vi "Try Match Response.vi"(8 "error in":errorcluster, 10 "ICAN CC Frame":refnum<class "ICAN CC Frame.lvclass">, 11 "Block Upload Transfer in":refnum<class "Block Upload Sub-Block Transfer.lvclass">) -> (0 "error out":errorcluster, 2 "Match":bool, 3 "SDO Transfer out":refnum<class "SDO Transfer.lvclass">)   [LabVIEW 2020, in "CANopen.lvlib" / "SDO Manager.lvlib" / "Block Upload Sub-Block Transfer.lvclass"]
uses:
  Block Upload Sub-Block Transfer.lvclass
  D:/git/CANopen-LabVIEW/source/SDO/SDO Manager/SDO Transfer/SDO Transfer.lvclass
  SDO Transfer/SDO Transfer.lvclass
  HAL/Source/Interfaces/ICAN CC Frame/ICAN CC Frame.lvclass
  D:/git/HAL/Source/Interfaces/IMessage/IMessage.lvclass
  SDO Transfer/SDO Transfer.lvclass/SDO Transfer.ctl
  Block Upload Sub-Block Transfer.lvclass/Block Upload Sub-Block Transfer.ctl
  Block Upload End Transfer/Block Upload End Transfer.lvclass
  HAL/Source/Interfaces/ICommunicate/ICommunicate.lvclass
  CANopen Message/CANopen Message.lvclass
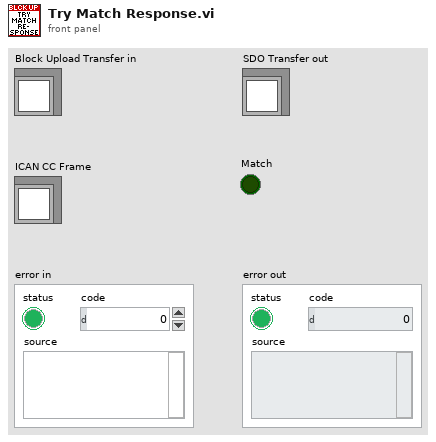
[diagram p1: front panel]
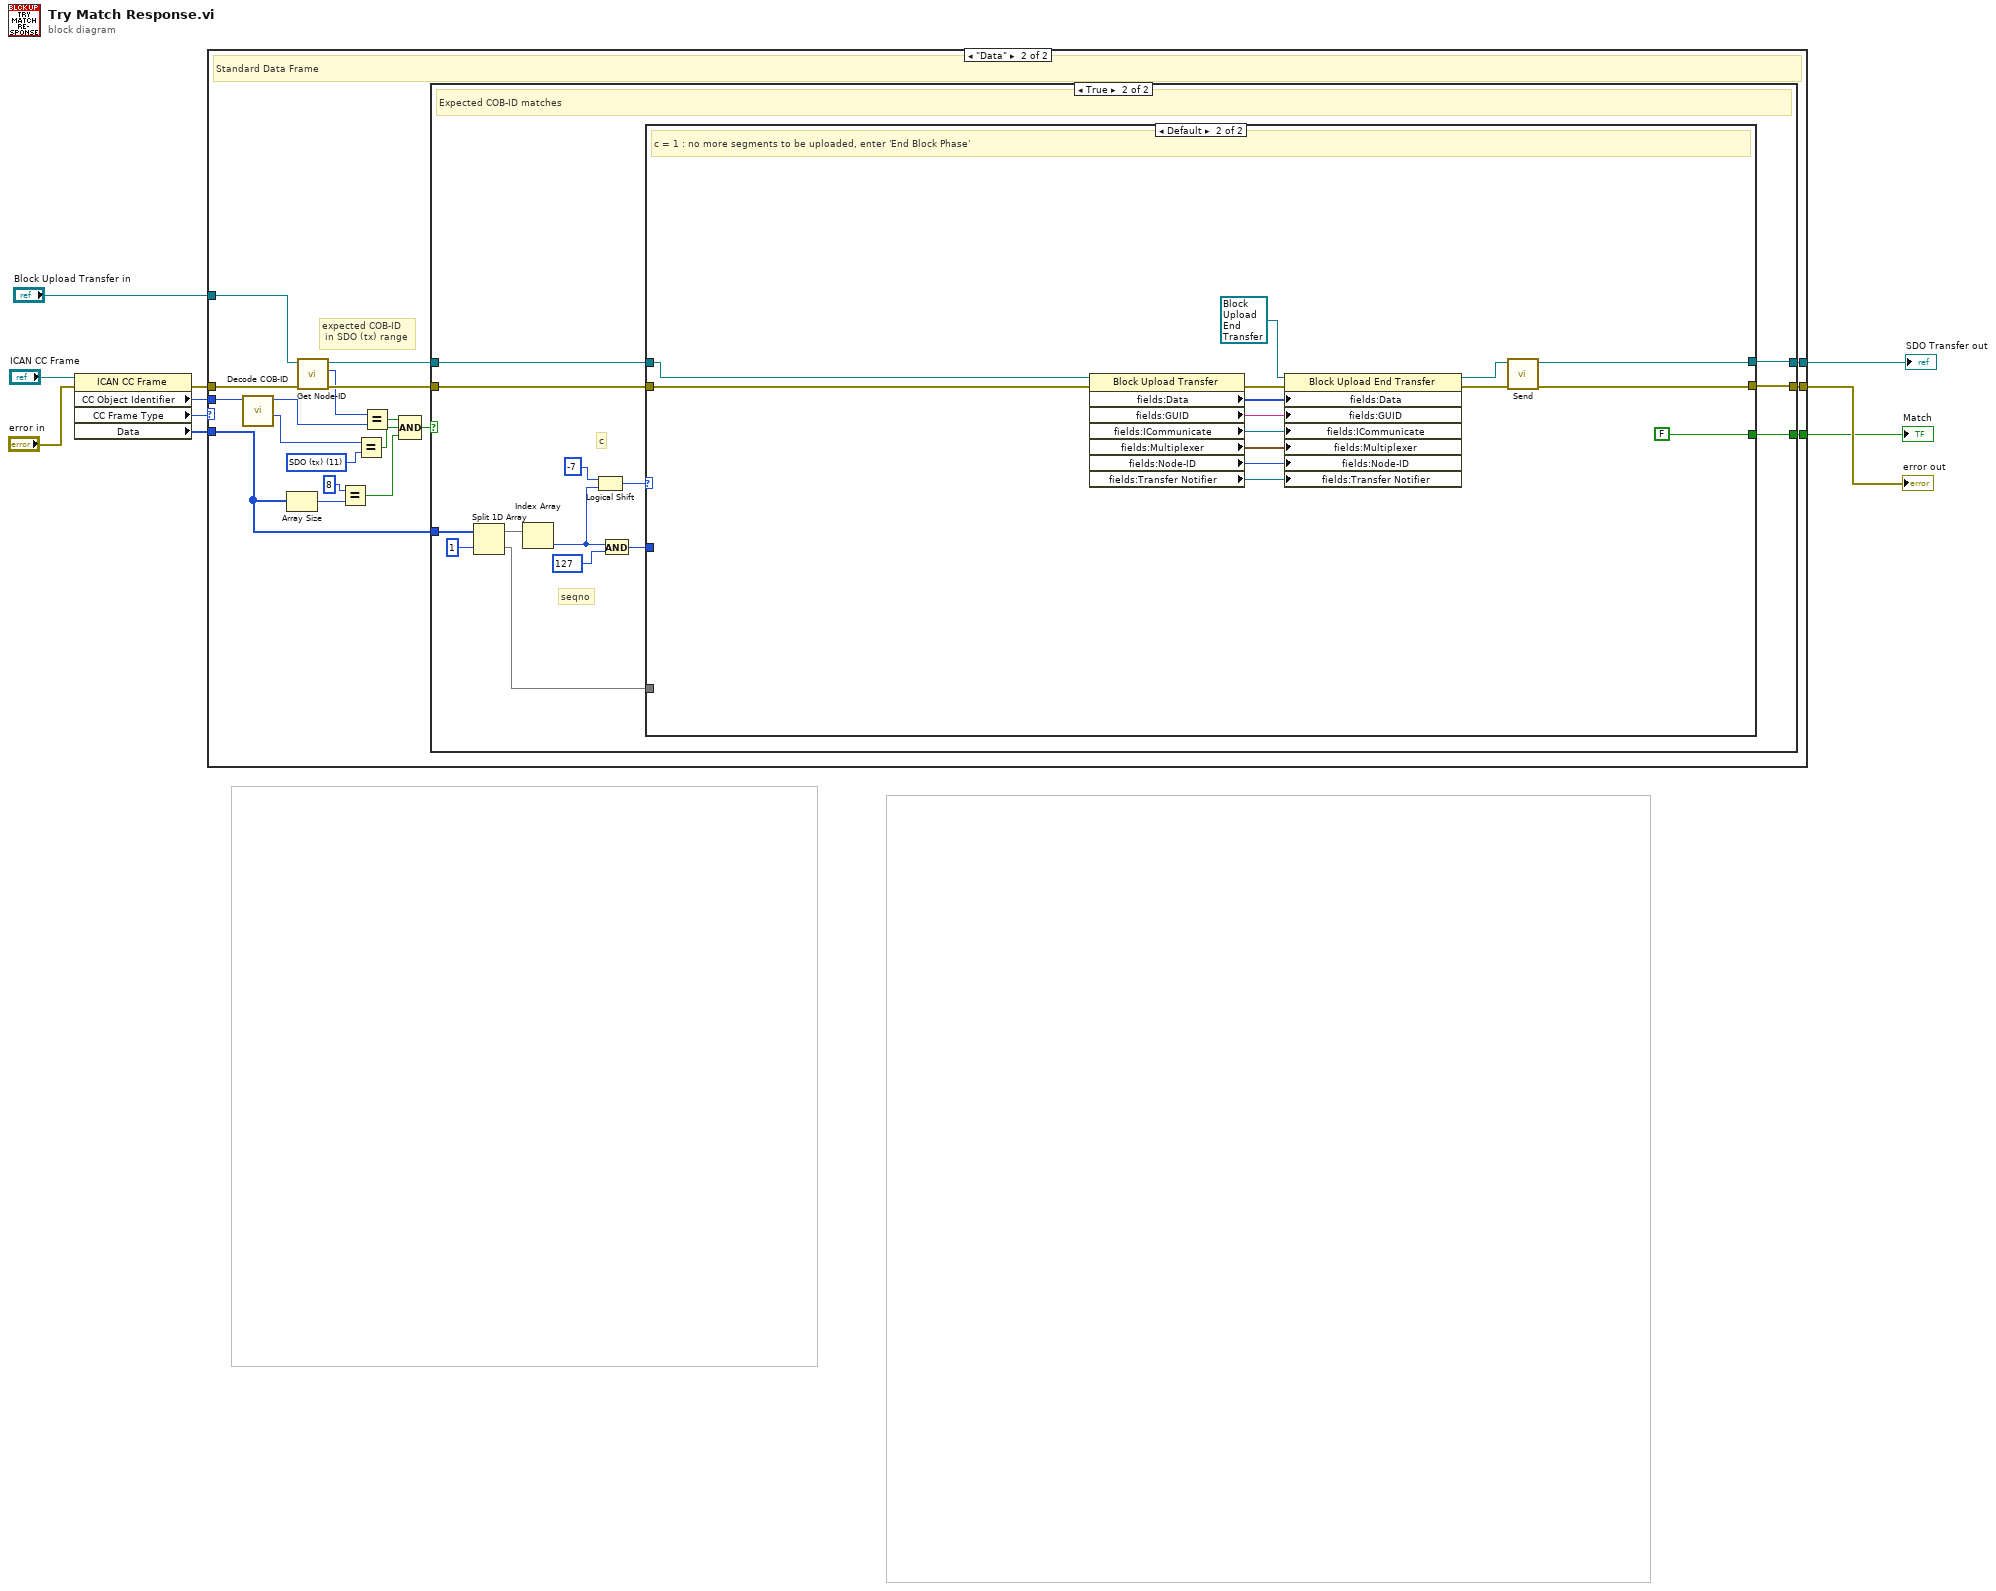
[diagram p0: block diagram]
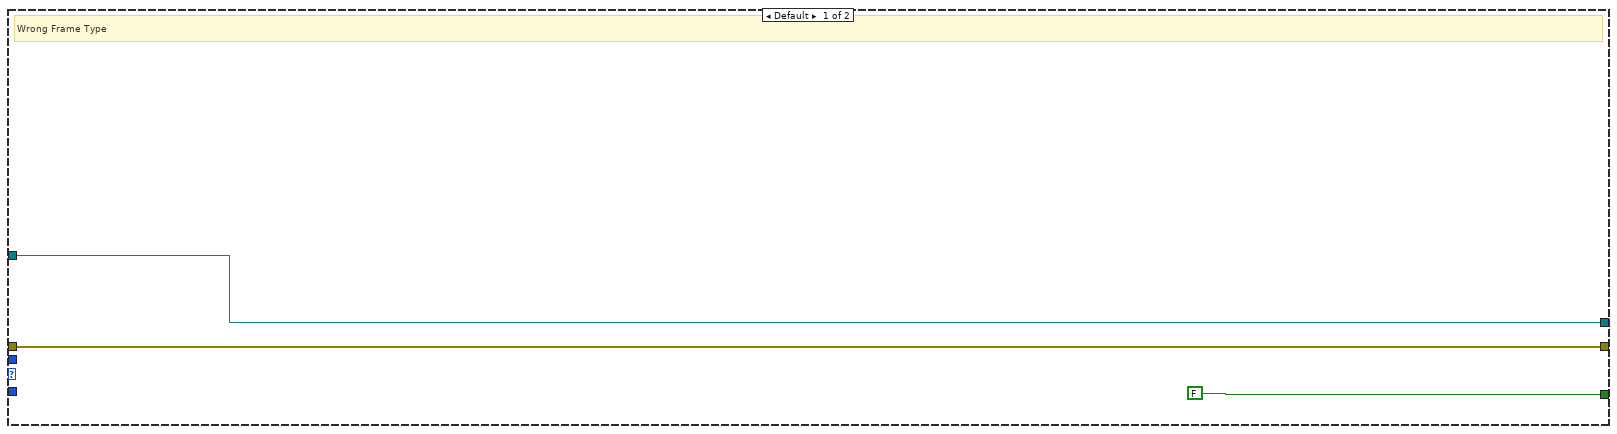
[diagram p2: hidden frame]
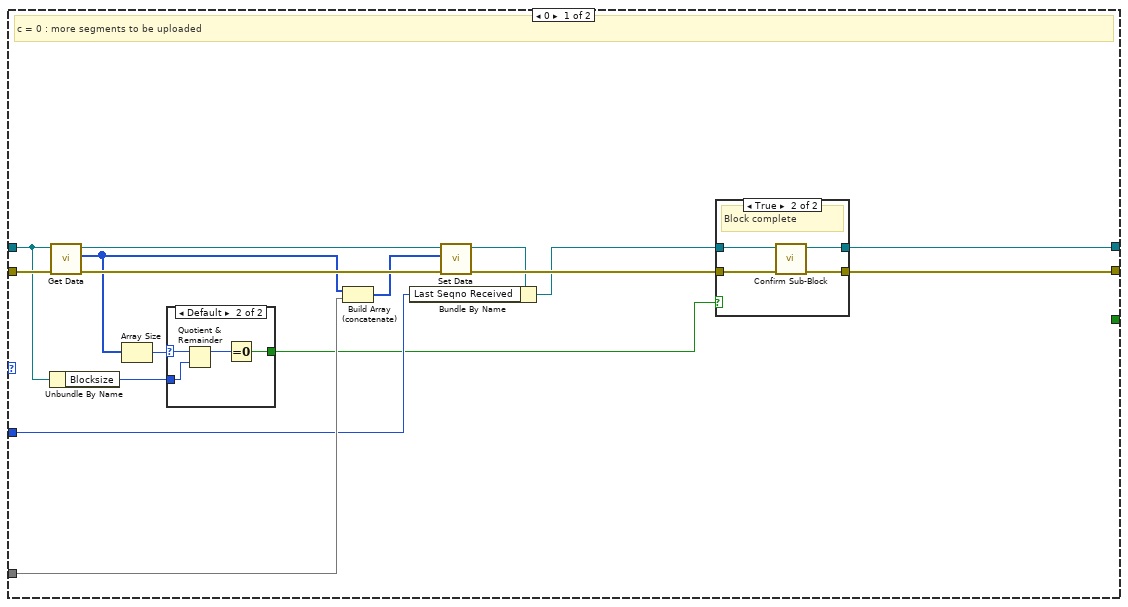
[diagram p4: hidden frame]
diagram:
  n1 = property class="ICAN CC Frame"(reference="ICAN CC Frame", error in="error in") -> (error out=w9:errorcluster, "CC Object Identifier"=w8:u32, "CC Frame Type"=w6:enum8{"Data", "Remote", "Error", "Overload"}, "Data"=w7:u8[])  [unwired: 1 out]
  n2 = case shown="\"Data\"" w6 {
    tunnel: w9 -> [w12 w32]
    tunnel: "Block Upload Transfer in" -> [w11 w31]
    tunnel: [w11 w28] -> w2
    tunnel: [w12 w27] -> w10
    tunnel: [FALSE w26] -> w1
    tunnel: w8 -> [_ w25]
    tunnel: w7 -> [_ w14]
    frame Default {
      # "Wrong Frame Type"
    }
    frame "Data" {
      w22 = u8 11 items=["NMT"=0, "EMCY/SYNC"=1, "TIME"=2, "PDO1 (tx)"=3, "PDO1 (rx)"=4, "PDO2 (tx)"=5, "PDO2 (rx)"=6, "PDO3 (tx)"=7, "PDO3 (rx)"=8, "PDO4 (tx)"=9, "PDO4 (rx)"=10, "SDO (tx)"=11, "SDO (rx)"=12, "NMT error control"=14] ("Function Code")
      # "expected COB-ID\n in SDO (tx) range"
      # "Standard Data Frame"
      n3 = call "Decode COB-ID.vi"("COD-ID"=w25) -> ("Function Code"=w21:u8, "Node-ID"=w24:u8)  [unwired: 9 in]
      n4 = Array Size(array=w14) -> (size(s)=w20:i32)
      n5 = call "Get Node-ID.vi"("error in"=w32, "SDO Transfer in"=w31) -> ("error out"=w29:errorcluster, "Node-ID"=w23:u8, "SDO Transfer out"=w30:refnum<class "Block Upload Sub-Block Transfer.lvclass">)  [unwired: 7 in]
      n6 = Equal?(x=8, y=w20) -> (x = y?=w15:bool)
      n7 = Equal?(x=w21, y=w22) -> (x = y?=w16:bool)
      n8 = Equal?(x=w23, y=w24) -> (x = y?=w17:bool)
      n9 = Compound Arithmetic op=AND(w17, w16, w15) -> (w18:bool)
      n10 = case shown="True" w18 {
        tunnel: w30 -> [w34 w47]
        tunnel: w29 -> [w33 w46]
        tunnel: [w34 w42] -> w28
        tunnel: [w33 w43] -> w27
        tunnel: w14 -> [_ w44]
        tunnel: [_ w41] -> w26
        frame False {
        }
        frame True {
          # "seqno"
          # "c"
          # "Expected COB-ID matches"
          n11 = Split 1D Array(array=w44, index=1) -> (first subarray=w38:u8[], second subarray=w39:u8[])
          n12 = Index Array(array=w38) -> (element=w36:u8)  [unwired: 1 in]
          n13 = Logical Shift(y=i16 -7, x=w36) -> (x << y=w45:u8)
          n14 = And(x=w36, y=u8 127 ("seqno")) -> (x .and. y?=w35:u8)
          n15 = case shown="Default" w45 {
            tunnel: w47 -> [w62 w84]
            tunnel: w46 -> [w64 w87]
            tunnel: [w50 w75] -> w42
            tunnel: [w52 w77] -> w43
            tunnel: [_ FALSE] -> w41
            tunnel: w39 -> [w54 _]
            tunnel: w35 -> [w53 _]
            frame 0 {
              # "c = 0 : more segments to be uploaded"
              n16 = Unbundle By Name(w62) -> ("Blocksize"=w60:u8)
              n17 = call "Get Data.vi"("error in"=w64, "SDO Transfer in"=w62) -> ("error out"=w63:errorcluster, "Data"=w56:u8[], "SDO Transfer out"=w58:refnum<class "Block Upload Sub-Block Transfer.lvclass">)  [unwired: 7 in]
              n18 = Array Size(array=w56) -> (size(s)=w61:i32)
              n19 = case shown="Default" w61 {
                selector: w61 -> [_ w74]
                tunnel: w60 -> [_ w73]
                tunnel: [_ w71] -> w49
                frame 0 {
                }
                frame Default {
                  n20 = Quotient & Remainder(x=w74, y=w73) -> (x-y*floor(x/y)=w72:i32)  [unwired: 1 out]
                  n21 = Equal To 0?(x=w72) -> (x = 0?=w71:bool)
                }
              }
              n22 = Build Array (concatenate)(w56, w54) -> (w55:u8[])
              n23 = call "Set Data.vi"("error in"=w63, "Data"=w55, "SDO Transfer in"=w58) -> ("error out"=w59:errorcluster, "SDO Transfer out"=w57:refnum<class "Block Upload Sub-Block Transfer.lvclass">)  [unwired: 7 in]
              n24 = Bundle By Name(cluster=w57, "Last Seqno Received"=w53) -> (w51:refnum<class "Block Upload Sub-Block Transfer.lvclass">)
              n25 = case shown="True" w49 {
                tunnel: w59 -> [w66 w70]
                tunnel: [w66 w69] -> w52
                tunnel: w51 -> [w65 w68]
                tunnel: [w65 w67] -> w50
                frame False {
                  # "Block incomplete"
                }
                frame True {
                  # "Block complete"
                  n26 = call "Confirm Sub-Block.vi"("error in"=w70, "Block Upload Transfer in"=w68) -> ("error out"=w69:errorcluster, "Block Upload Transfer out"=w67:refnum<class "Block Upload Sub-Block Transfer.lvclass">)  [unwired: 8 in]
                }
              }
            }
            frame Default {
              # "c = 1 : no more segments to be uploaded, enter 'End Block Phase'"
              n27 = property class="Block Upload Transfer"(reference=w84, error in=w87) -> (error out=w85:errorcluster, "fields:Data"=w83:u8[], "fields:GUID"=w82:string, "fields:ICommunicate"=w81:refnum<class "ICommunicate.lvclass">, "fields:Multiplexer"=w80:cluster{"Index":u16, "Sub-Index":u8}, "fields:Node-ID"=w79:u8, "fields:Transfer Notifier"=w78:refnum<notifier>)  [unwired: 1 out]
              n28 = property class="Block Upload End Transfer"(reference=refnum<class "Block Upload End Transfer.lvclass"> refnum ("CANopen.lvlib:SDO Manager.lvlib:Block Upload End Transfer"), error in=w85, "fields:Data"=w83, "fields:GUID"=w82, "fields:ICommunicate"=w81, "fields:Multiplexer"=w80, "fields:Node-ID"=w79, "fields:Transfer Notifier"=w78) -> (reference out=w76:refnum<class "Block Upload End Transfer.lvclass">, error out=w86:errorcluster)
              n29 = call-dynamic "Send.vi"("error in"=w86, "Block Upload End Transfer in"=w76) -> ("error out"=w77:errorcluster, "Block Upload End Transfer out"=w75:refnum<class "Block Upload End Transfer.lvclass">)  [unwired: 8 in]
            }
          }
        }
      }
    }
  }
  "SDO Transfer out" <- w2
  "error out" <- w10
  "Match" <- w1
